vi "testMap.vi"() -> (0 "error out":errorcluster)   [LabVIEW 2019, in "AssertionTest.lvlib" / "AssertCount.lvlib"]
uses:
  AssertCount.lvlib
  Assertion/Assertion.lvlib
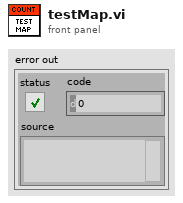
[diagram p1: front panel]
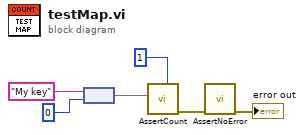
[diagram p0: block diagram]
diagram:
  n1 = node("My key" ("key"), 0 ("value")) -> (w4:map{string, i32})
  n2 = call "AssertCount.vi"("Expected"=1, "Haystack"=w4) -> ("error out"=w2:errorcluster)  [unwired: 9 in]
  n3 = call "AssertNoError.vi"("error in (no error)"=w2) -> ("error out"=→"error out":errorcluster)  [unwired: 10 in]
